vi "[U8] to [BOOL].vi"(1 "[U8]":u8[][](array[numeric])) -> (0 "[BOOL]":bool[][](array[boolean]))   [LabVIEW 2026, in "GoL.lvlib"]
uses:
  GoL.lvlib
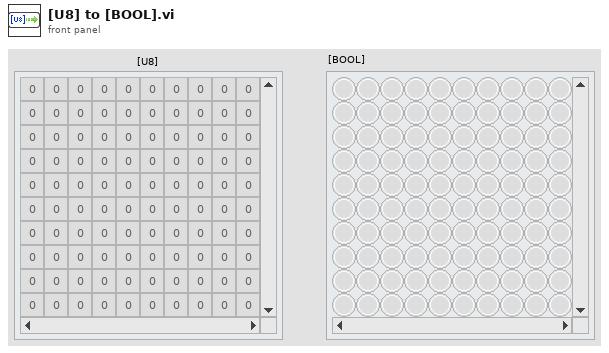
[diagram p1: front panel]
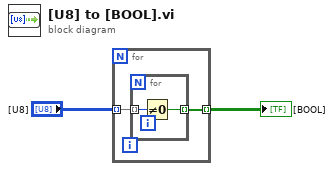
[diagram p0: block diagram]
diagram:
  n1 = for {
    tunnel: "[U8]" -> [w4] mode=indexing
    tunnel: [w3] -> w1 mode=indexing
    n2 = for {
      tunnel: w4 -> [w6] mode=indexing
      tunnel: [w5] -> w3 mode=indexing
      n3 = Not Equal To 0?(x=w6) -> (x != 0?=w5:bool)
    }
  }
  "[BOOL]" <- w1
